vi "oath2_auth_url-pkce.vi"(8 "error in (no error)":errorcluster, 9 "code_challenege_method":T1=enum."sha256", 10 "challenge":string, 11 "client_id":string) -> (0 "error out":errorcluster, 3 "auth_url":string)   [LabVIEW 2015, in "lv-dropbox.lvlib"]
uses:
  lv-dropbox.lvlib
  _controls/code_challenge_method.ctl
  private/cryptography/cryptography.lvlib
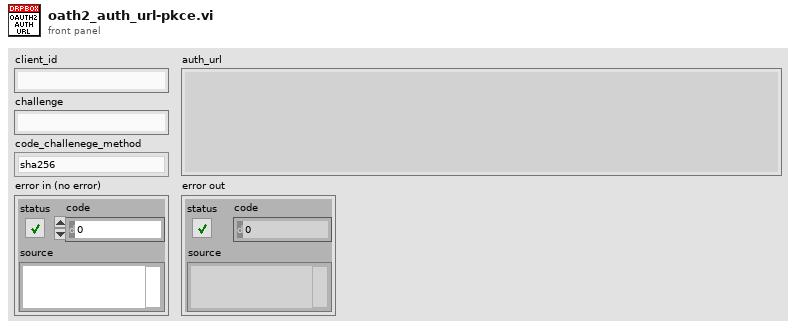
[diagram p1: front panel]
types:
  T1 = typedef "lv-dropbox.lvlib/code_challenge_method.ctl" = enum16{"<challenge_method>", "plain", "sha256"}
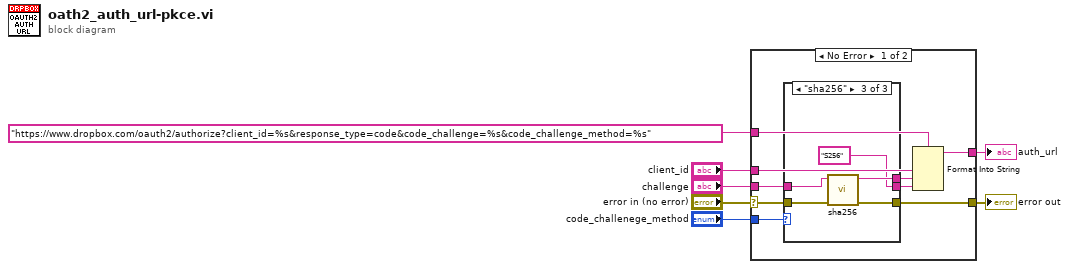
[diagram p0: block diagram]
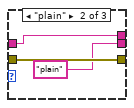
[diagram p3: hidden frame]
diagram:
  n1 = case shown="No Error" "error in (no error)" {
    selector: "error in (no error)" -> [w13 w26]
    tunnel: [w11 w26] -> w5
    tunnel: "https://www.dropbox.com/oauth2/authorize?client_id=%s&response_type=code&code_challenge=%s&code_challenge_method=%s" ("url") -> [w8 _]
    tunnel: "client_id" -> [w16 _]
    tunnel: "challenge" -> [w14 _]
    tunnel: [w12 _] -> w2
    tunnel: "code_challenege_method" -> [w10 _]
    frame No Error {
      n2 = case shown="\"sha256\"" w10 {
        tunnel: [_ w20 w25] -> w15
        tunnel: w14 -> [_ w20 w24]
        tunnel: w13 -> [w17 w19 w23]
        tunnel: [w17 w19 w22] -> w11
        tunnel: [_ "plain" ("url") "S256" ("url")] -> w9
        frame Default {
        }
        frame "plain" {
        }
        frame "sha256" {
          n3 = call "sha256.vi"("error in (no error)"=w23, "data_decoded"=w24) -> ("error out"=w22:errorcluster, "data_encoded"=w25:string)  [unwired: 8 in]
        }
      }
      n4 = Format Into String(format string=w8, w16, w15, w9) -> (resulting string=w12:string)  [unwired: 2 in, 1 out]
    }
    frame Error {
    }
  }
  "error out" <- w5
  "auth_url" <- w2
